vi "Drive Test.vi"() -> ()   [LabVIEW 2014]
panel:
  in  "Slow":bool
  in  "Reset":bool
  in  "Turn":dbl format="%#_13g"
  in  "Forward/Backward":dbl
  in  "Strafe":dbl
  out "Distance (ft)":dbl
  in  "stop":bool
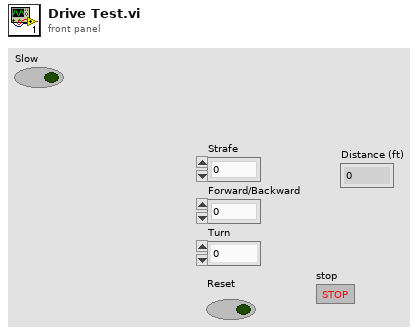
[diagram p1: front panel]
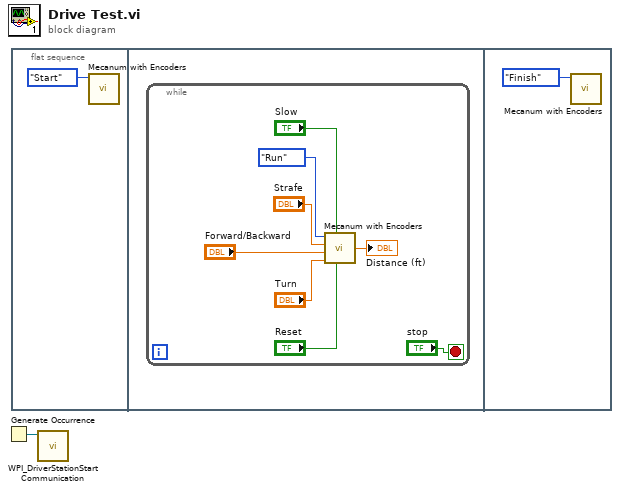
[diagram p0: block diagram]
diagram:
  n1 = Generate Occurrence() -> (w1:refnum<k4>)
  n2 = flat-sequence {
    frame #0 {
      n3 = call "Mecanum with Encoders.vi"("Mode"=enum8{"Start", "Run", "Finish"}."Start") -> ()  [unwired: 5 in, 1 out]
    }
    frame #1 {
      n4 = while {
        stop <- "stop" stop-if-true
        n5 = call "Mecanum with Encoders.vi"("Reset"="Reset", "Slow"="Slow", "Turn"="Turn", "Forward/Backward"="Forward/Backward", "Strafe"="Strafe", "Mode"=enum8{"Start", "Run", "Finish"}."Run") -> ("Distance (ft)"=→"Distance (ft)":dbl)
      }
    }
    frame #2 {
      n6 = call "Mecanum with Encoders.vi"("Mode"=enum8{"Start", "Run", "Finish"}."Finish") -> ()  [unwired: 5 in, 1 out]
    }
  }
  n7 = call <vilib>:"WPI_DriverStationStart Communication.vi"("occurrence"=w1) -> ()  [unwired: 11 in]
